vi "timestampOffset.vi"(10 "Reference Time":timestamp) -> (2 "Timestamp Offset":i64)   [LabVIEW 2013]
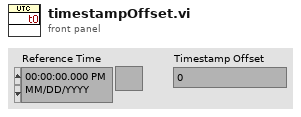
[diagram p1: front panel]
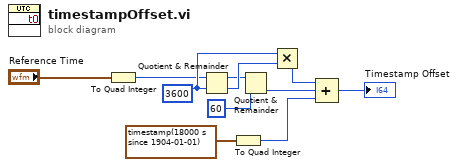
[diagram p0: block diagram]
diagram:
  w5 = i64 3600 ("y")
  n1 = To Quad Integer(1:"Reference Time") -> (0:w3:i64)
  n2 = Quotient & Remainder(x=w3, y=w5) -> (x-y*floor(x/y)=w2:i64, floor(x/y)=w6:i64)
  n3 = To Quad Integer(1:timestamp(18000 s since 1904-01-01) ("current time")) -> (0:w8:i64)
  n4 = Quotient & Remainder(x=w2, y=i64 60) -> (floor(x/y)=w9:i64)  [unwired: 1 out]
  n5 = Multiply(x=w5, y=w6) -> (x*y=w10:i64)
  n6 = Compound Arithmetic op=ADD(w10, w9, w8) -> (→"Timestamp Offset":i64)
